vi "apply txt extension to file name.vi"(1 "File name (excluding extension)":string) -> (0 "File name (with .txt extension)":string)   [LabVIEW 2020, in "text_file.lvlib"]
doc: "Applies (appends) the \".txt\" file extension to a file name."
uses:
  text_file.lvlib
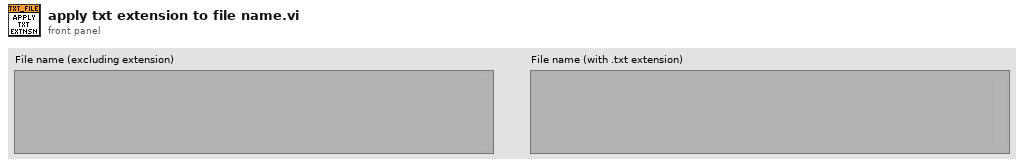
[diagram p1: front panel]
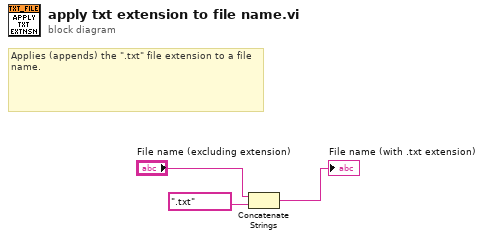
[diagram p0: block diagram]
diagram:
  # "Applies (appends) the \".txt\" file extension to a file name."
  n1 = Concatenate Strings("File name (excluding extension)", ".txt" ("string")) -> (→"File name (with .txt extension)":string)
